vi "CTRE_PigeonIMU_SetTempCompensationEnable.vi"(8 "error in (no error)":errorcluster, 10 "Enable?":bool=TRUE, 11 "PigeonIMUDevRef":T1={"DeviceStatus"={"status"=FALSE, "code"=0, "source"=""}, "Device Number"=0, "Type"=352321536, "Device ID"=0} {"Type" items=["CAN"=352321536, "TalonSRX"=33554432]}) -> (0 "error out":errorcluster, 3 "PigeonIMUDevRef Out":T1={"DeviceStatus"={"status"=FALSE, "code"=0, "source"=""}, "Device Number"=0, "Type"=352321536, "Device ID"=0} {"Type" items=["CAN"=352321536, "TalonSRX"=33554432]})   [LabVIEW 2016]
uses:
  <vilib>/Rock Robotics/WPI/ThirdParty/Sensors/Pigeon/CTRE_PigeonIMU_DeviceRef.ctl
  <vilib>/Rock Robotics/WPI/ThirdParty/Sensors/Pigeon/CTRE_PigeonIMU_ConnectionType.ctl
  <vilib>/Rock Robotics/WPI/ThirdParty/Sensors/Pigeon/CTRE_PigeonIMU_TareType.ctl
  <vilib>/Rock Robotics/WPI/ThirdParty/Sensors/Pigeon/CTRE_PigeonIMU_Params.ctl
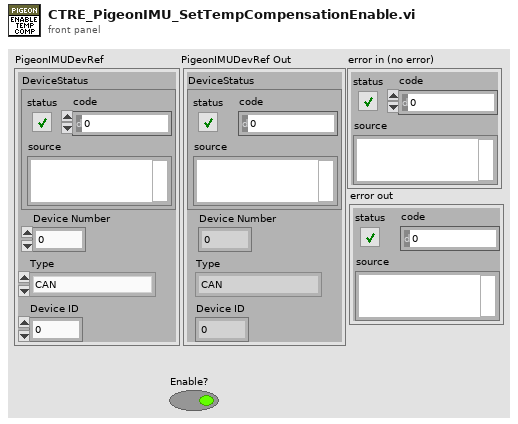
[diagram p1: front panel]
types:
  T1 = typedef "CTRE_PigeonIMU_DeviceRef.ctl" = cluster{"DeviceStatus":errorcluster, "Device Number":u8, "Type":T2, "Device ID":u32}
  T2 = typedef "CTRE_PigeonIMU_ConnectionType.ctl" = u32
  T3 = typedef "CTRE_PigeonIMU_Params.ctl" = u8
  T4 = typedef "CTRE_PigeonIMU_TareType.ctl" = u8
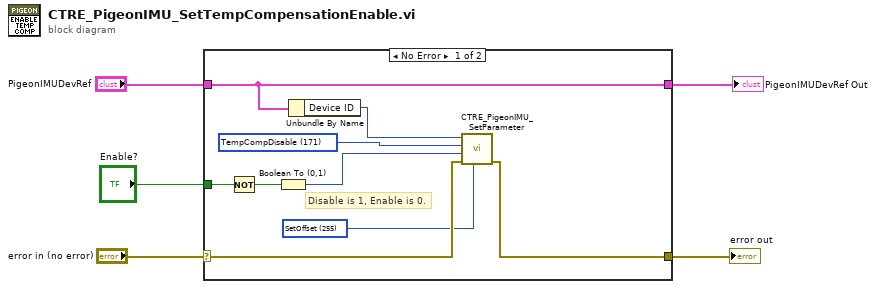
[diagram p0: block diagram]
diagram:
  n1 = case shown="No Error" "error in (no error)" {
    selector: "error in (no error)" -> [w12 w15]
    tunnel: [w11 w15] -> w4
    tunnel: [w14 w16] -> w2
    tunnel: "PigeonIMUDevRef" -> [w14 w16]
    tunnel: "Enable?" -> [w8 _]
    frame No Error {
      w9 = T3 171 items=["YawOffset"=160, "CompassOffset"=161, "BetaGain"=162, "Reserved163"=163, "GyroNoMotionCal"=164, "EnterCalibration"=165, "FusedHeadingOffset"=166, "StatusFrameRate"=169, "AccumZ"=170, "TempCompDisable"=171] ("Parameter")
      w10 = T4 255 items=["SetValue"=0, "AddOffset"=1, "MatchCompass"=2, "SetOffset"=255] ("TareType")
      # "Disable is 1, Enable is 0."
      n2 = Not(x=w8) -> (.not. x?=w6:bool)
      n3 = Boolean To (0,1)(Boolean=w6) -> (0, 1=w7:i16)
      n4 = Unbundle By Name(w14) -> ("Device ID"=w13:u32)
      n5 = call <vilib>:"CTRE_PigeonIMU_SetParameter.vi"("TareType"=w10, "error in (no error)"=w12, "Value"=w7, "Parameter"=w9, "Device ID (0)"=w13) -> ("error out"=w11:errorcluster)  [unwired: 5 in, 1 out]
    }
    frame Error {
    }
  }
  "PigeonIMUDevRef Out" <- w2
  "error out" <- w4
